vi "NumIntegrate_Rkf45_Mat_X_U.vi"(5 "Func_X_U_Extra":T1, 6 "MaxError":dbl=1e-06, 7 "PassedData":variant, 8 "dT_Seconds":dbl, 10 "U":T2, 11 "X":T2) -> (0 "Error":bool, 1 "IterationCount":i32, 3 "Return X":T2)   [LabVIEW 2019, in "Trajectory_Library.lvlib"]
doc: "Performs adaptive RKF45 integration of dx/dt = f(x, u) for dt, as described in https://en.wikipedia.org/wiki/Runge%E2%80%93Kutta%E2%80%93Fehlberg_method\n\nInputs:\n - Func_X_U_Extra -- A strictly typed LabVIEW reference to a function to integrate as a function of matrix X, U, and the extra passed data\n - PassedData -- This is a variant that can be used to pass additional data to the function if needed. The data must be packed into the variant in the specific way expected by the function.\n - X -- X input matrix\n - U -- U input matrix.\n - dT -- The time over which to integrate\n - maxError -- The maximum acceptable truncation error. Usually a small number like 1e-6.\n\nOutputs:\n - Return X -- the integration of dx/dt = f(x, u) for dt.\n - Error -- If TRUE, an error occured.\n - Iteration Count -- The number of times the integration iterated to reach the desired maxError."
uses:
  Trajectory_Library.lvlib
  <vilib>/Analysis/Matrix/Datatypes/RealMatrix.ctl
  <vilib>/Analysis/Matrix/NI_Matrix.lvlib
  TypeDef/CALLBACK_FUNC_TYPE.ctl
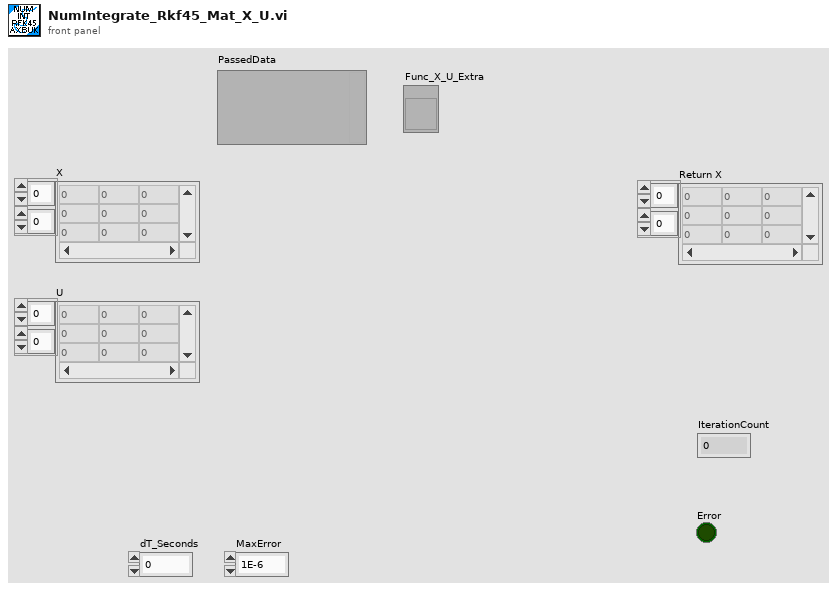
[diagram p1: front panel]
types:
  T1 = typedef "Trajectory_Library.lvlib/CALLBACK_FUNC_TYPE.ctl" = refnum<vi>
  T2 = typedef "NI_Matrix.lvlib/RealMatrix.ctl" = dbl[][]
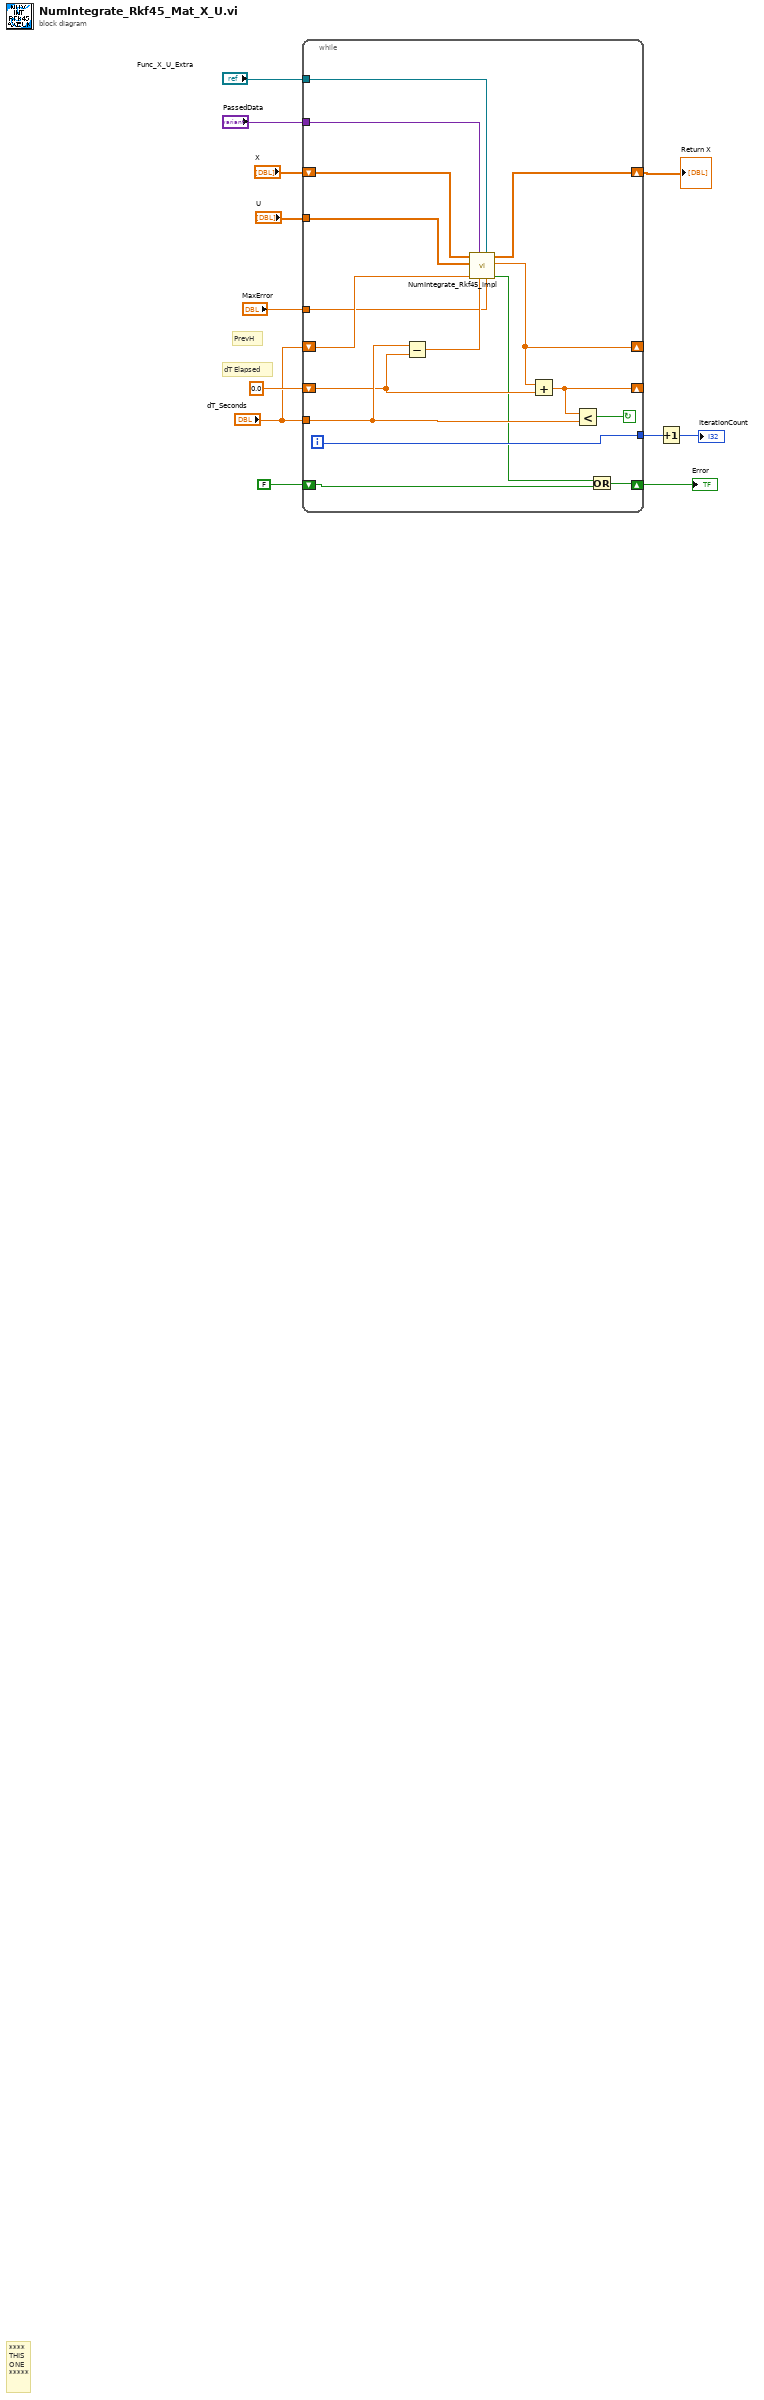
[diagram p0: block diagram]
diagram:
  # "PrevH"
  # "dT Elapsed"
  # "****\nTHIS\nONE\n*****"
  n1 = while {
    shift-right: [w21] -> _
    shift-left: 0.0 -> [w20]
    tunnel: "dT_Seconds" -> [w24]
    shift-right: [w19] -> _
    shift-left: "dT_Seconds" -> [w25]
    shift-right: [w27] -> w8
    shift-left: "X" -> [w28]
    tunnel: "U" -> [w26]
    tunnel: "MaxError" -> [w22]
    tunnel: [w18] -> w5
    tunnel: "Func_X_U_Extra" -> [w17]
    tunnel: "PassedData" -> [w16]
    shift-right: [w15] -> w1
    shift-left: FALSE -> [w14]
    i -> [w18]
    stop <- w29 continue-if-true
    n2 = Subtract(x=w24, y=w20) -> (x-y=w23:dbl)
    n3 = call "NumIntegrate_Rkf45_impl.vi"("MaxTruncError"=w22, "Func_X_U_Extra"=w17, "dT_Remaining"=w23, "PassedData"=w16, "InitialH"=w25, "U"=w26, "X"=w28) -> ("Error"=w13:bool, "H"=w19:dbl, "NewX"=w27:T2)  [unwired: 1 in, 1 out]
    n4 = Add(x=w19, y=w20) -> (x+y=w21:dbl)
    n5 = Less?(x=w21, y=w24) -> (x < y?=w29:bool)
    n6 = Or(x=w13, y=w14) -> (x .or. y?=w15:bool)
  }
  "Return X" <- w8
  "Error" <- w1
  n7 = Increment(x=w5) -> (x+1=→"IterationCount":i32)
